vi "Actor Core.vi"(8 "error in":errorcluster, 11 "HIJ 4 Aligment Cams Launcher in":refnum<class "HIJ 4 Aligment Cams Launcher.lvclass">) -> (0 "error out":errorcluster, 3 "Actor out":refnum<class "Actor.lvclass">)   [LabVIEW 2014, in "HIJ 4 Alignment Cams App.lvlib" / "HIJ 4 Aligment Cams Launcher.lvclass"]
doc: "(<B>Filename</B>: Actor Framework.lvlib:Actor.lvclass:Actor Core.vi)\n\nReceives messages to the actor, reacts to them, and initiates any error handling that may shut the actor down.\n\nDescendant classes may override this VI to append parallel tasks for the actor to complete while it handles messages. Overrides use the Call Parent Method node."
uses:
  HIJ 4 Aligment Cams Launcher.lvclass
  <vilib>/ActorFramework/Actor/Actor.lvclass
  <vilib>/userdefined/High Color/IMAQdx.ctl
  HIJ 4 Alignment Cams App/HIJ 4 Alignment Cams App.lvclass
  HIJ Vision Launcher/HIJ Vision Launcher/HIJ Vision Launcher.lvclass/HIJ Vision Launcher.ctl
  Shared Code/Viewable Actor/ViewableActor/ViewableActor.lvclass/ViewableActor.ctl
  HIJ 4 Alignment Cams App/HIJ 4 Alignment Cams App.lvclass/HIJ 4 Alignment Cams App.ctl
  <vilib>/ActorFramework/Actor/Actor.lvclass/Actor.ctl
  <vilib>/ActorFramework/Message Enqueuer/Message Enqueuer.lvclass/Message Enqueuer.ctl
  HIJ 4 Aligment Cams Launcher Messages/Set Sart Cameras Msg/Set Sart Cameras Msg.lvclass/Set Sart Cameras Msg.ctl
  HIJ Vision Launcher/HIJ Vision Launcher/Read HIJ Vision Camera App.vi
  HIJ Vision Launcher/HIJ Vision Launcher/Read Cmd Parameters.vi
  Shared Code/Viewable Actor/ViewableActor/Read Config URL.vi
  HIJ 4 Alignment Cams App/Write Start Camera 4.vi
  HIJ 4 Alignment Cams App/Write Start Camera 3.vi
  HIJ 4 Alignment Cams App/Write Start Camera 2.vi
  HIJ Vision Launcher/HIJ Vision Launcher/Write HIJ Vision Camera App.vi
  <vilib>/ActorFramework/Message Enqueuer/Init from Existing Queue.vi
  <vilib>/ActorFramework/Message Enqueuer/Enqueue.vi
  <vilib>/Utility/config.llb/Read Key (String).vi
  <vilib>/Utility/config.llb/Write Key (String).vi
  <vilib>/ActorFramework/Message Priority Queue/Priority Enqueue.vi
  Shared Code/Viewable Actor/ViewableActor/ViewableActor.lvclass
  <vilib>/ActorFramework/Message Enqueuer/Message Enqueuer.lvclass
  HIJ 4 Aligment Cams Launcher Messages/Set Sart Cameras Msg/Set Sart Cameras Msg.lvclass
  <vilib>/ActorFramework/Stop Msg/Stop Msg.lvclass
  HIJ Vision Launcher/HIJ Vision Launcher/HIJ Vision Launcher.lvclass
  <vilib>/Utility/config.llb/NI_LVConfig.lvlib
panel:
  in  "Camera 2":T1="dummy"
  in  "Camera 3":T1="dummy"
  in  "Main Camera 4":T1="dummy"
  in  "RUN_STOP":bool
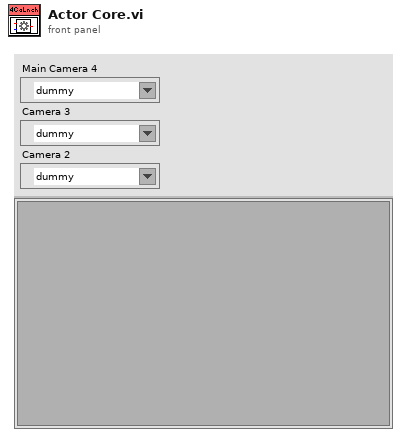
[diagram p1: front panel]
types:
  T1 = typedef "IMAQdx.ctl" = refnum<k21>
  T2 = typedef "NI_LVConfig.lvlib/Config Data RefNum.ctl" = refnum<k1>
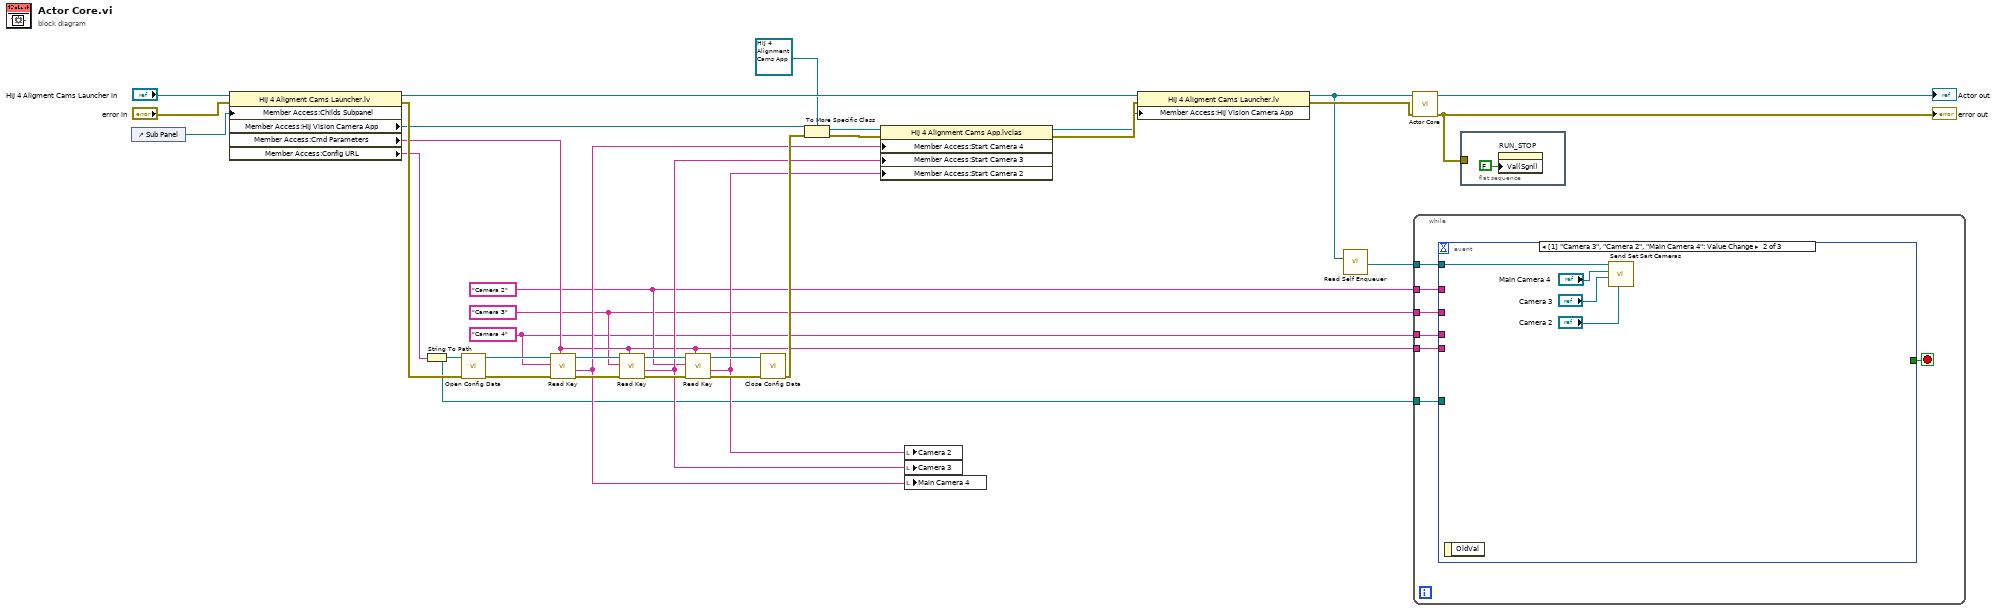
[diagram p0: block diagram]
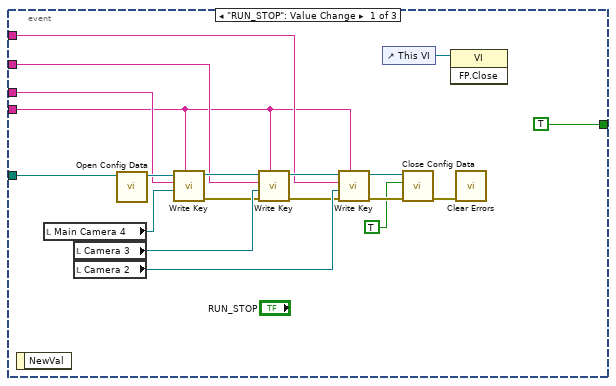
[diagram p2: hidden frame]
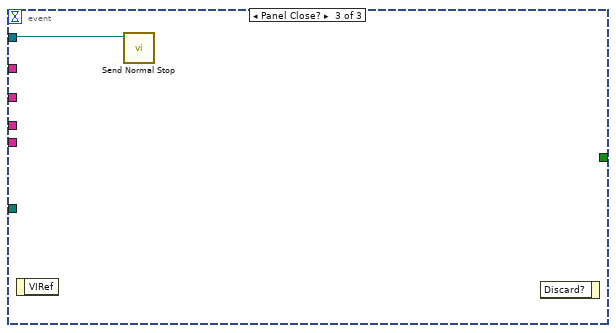
[diagram p3: hidden frame]
diagram:
  w10 = "Camera 2" ("key")
  w9 = "Camera 3" ("key")
  w8 = "Camera 4" ("key")
  n1 = control-ref of="Sub Panel"() -> (w29:refnum<vi>)
  n2 = property class="HIJ 4 Aligment Cams Launcher.lv"(reference="HIJ 4 Aligment Cams Launcher in", error in="error in", "Member Access:Childs Subpanel"=w29) -> (reference out=w30:refnum<class "HIJ 4 Aligment Cams Launcher.lvclass">, error out=w33:errorcluster, "Member Access:HIJ Vision Camera App"=w4:refnum<class "ViewableActor.lvclass">, "Member Access:Cmd Parameters"=w11:string, "Member Access:Config URL"=w28:string)
  n3 = String To Path(string=w28) -> (path=w16:path)
  n4 = call <vilib>:"Open Config Data.vi"("error in (no error)"=w33, "configuration file path"=w16) -> ("error out"=w27:errorcluster, "refnum"=w26:T2)  [unwired: 7 in, 1 out]
  n5 = call-poly <vilib>:"Read Key.vi"("section"=w11, "error in (no error)"=w27, "key"=w8, "refnum"=w26) -> ("error out"=w24:errorcluster, "value"=w19:string, "refnum out"=w25:T2)  [unwired: 4 in, 1 out]
  n6 = call-poly <vilib>:"Read Key.vi"("section"=w11, "error in (no error)"=w24, "key"=w9, "refnum"=w25) -> ("error out"=w22:errorcluster, "value"=w18:string, "refnum out"=w23:T2)  [unwired: 4 in, 1 out]
  n7 = call-poly <vilib>:"Read Key.vi"("section"=w11, "error in (no error)"=w22, "key"=w10, "refnum"=w23) -> ("error out"=w20:errorcluster, "value"=w17:string, "refnum out"=w21:T2)  [unwired: 4 in, 1 out]
  n8 = call <vilib>:"Close Config Data.vi"("error in (no error)"=w20, "refnum"=w21) -> ("error out"=w34:errorcluster)  [unwired: 8 in, 1 out]
  n9 = To More Specific Class(target class=refnum<class "HIJ 4 Alignment Cams App.lvclass"> refnum ("HIJ 4 Alignment Cams App.lvlib:HIJ 4 Alignment Cams App.lvclass"), reference=w4, error in=w34) -> (specific class reference=w1:refnum<class "HIJ 4 Alignment Cams App.lvclass">, error out=w3:errorcluster)
  n10 = property class="HIJ 4 Alignment Cams App.lvclas"(reference=w1, error in=w3, "Member Access:Start Camera 4"=w19, "Member Access:Start Camera 3"=w18, "Member Access:Start Camera 2"=w17) -> (reference out=w2:refnum<class "HIJ 4 Alignment Cams App.lvclass">, error out=w14:errorcluster)
  n11 = local write "Camera 2"(w17) -> ()
  n12 = local write "Camera 3"(w18) -> ()
  n13 = local write "Main Camera 4"(w19) -> ()
  n14 = property class="HIJ 4 Aligment Cams Launcher.lv"(reference=w30, error in=w14, "Member Access:HIJ Vision Camera App"=w2) -> (reference out=w12:refnum<class "HIJ 4 Aligment Cams Launcher.lvclass">, error out=w13:errorcluster)
  n15 = call <vilib>:"Read Self Enqueuer.vi"("Actor"=w12) -> ("Self Enqueuer"=w7:refnum<class "Message Enqueuer.lvclass">)  [unwired: 10 in]
  n16 = call-parent "Actor Core.vi"("error in"=w13, "HIJ Vision Launcher in"=w12) -> ("error out"=w6:errorcluster, "Actor out"=→"Actor out":refnum<class "Actor.lvclass">)  [unwired: 8 in]
  "error out" <- w6
  n17 = while {
    tunnel: w11 -> [w40]
    tunnel: w16 -> [w39]
    tunnel: w8 -> [w38]
    tunnel: w9 -> [w37]
    tunnel: w10 -> [w36]
    tunnel: w7 -> [w35]
    stop <- w41 stop-if-true
    n18 = event shown="[1] \"Camera 3\", \"Camera 2\", \"Main Camera 4\": Value Change" {
      selector: _ -> [_ _ _]
      dyn-events: _ -> [_ _ _]
      timeout: _ -> [_ _ _]
      tunnel: [TRUE _ _] -> w41
      tunnel: w40 -> [w43 _ _]
      tunnel: w39 -> [w48 _ _]
      tunnel: w38 -> [w46 _ _]
      tunnel: w37 -> [w45 _ _]
      tunnel: w36 -> [w44 _ _]
      tunnel: w35 -> [_ w64 w65]
      event "RUN_STOP": Value Change {
        n19 = event-data() -> ()  [unwired: 1 in, 1 out]
        n20 = local read "Main Camera 4"() -> (w53:T1)
        n21 = local read "Camera 3"() -> (w58:T1)
        n22 = local read "Camera 2"() -> (w59:T1)
        n23 = call <vilib>:"Open Config Data.vi"("configuration file path"=w48) -> ("refnum"=w47:T2)  [unwired: 8 in, 2 out]
        n24 = call-poly <vilib>:"Write Key.vi"("section"=w43, "value"=w53, "key"=w46, "refnum"=w47) -> ("error out"=w51:errorcluster, "refnum out"=w52:T2)  [unwired: 5 in, 1 out]
        n25 = call-poly <vilib>:"Write Key.vi"("section"=w43, "error in (no error)"=w51, "value"=w58, "key"=w45, "refnum"=w52) -> ("error out"=w56:errorcluster, "refnum out"=w57:T2)  [unwired: 4 in, 1 out]
        n26 = call-poly <vilib>:"Write Key.vi"("section"=w43, "error in (no error)"=w56, "value"=w59, "key"=w44, "refnum"=w57) -> ("error out"=w55:errorcluster, "refnum out"=w54:T2)  [unwired: 4 in, 1 out]
        n27 = control-ref of="This VI"() -> (w42:refnum<vi>)
        n28 = call <vilib>:"Close Config Data.vi"("error in (no error)"=w55, "write file if changed (T)"=TRUE, "refnum"=w54) -> ("error out"=w49:errorcluster)  [unwired: 7 in, 1 out]
        n29 = invoke class="VI" method="FP.Close"(reference=w42) -> ()  [unwired: 2 in, 3 out]
        n30 = call <vilib>:"Clear Errors.vi"("error in (no error)"=w49) -> ()  [unwired: 5 in, 2 out]
      }
      event Value Change {
        n31 = event-data() -> ()  [unwired: 1 in, 1 out]
        n32 = call "Send Set Sart Cameras.vi"("Camera 2"="Camera 2", "Camera 3"="Camera 3", "Main Camera 4"="Main Camera 4", "Message Enqueuer"=w64) -> ()  [unwired: 6 in, 2 out]
      }
      event Panel Close? {
        n33 = event-data() -> ()  [unwired: 1 in, 1 out]
        n34 = call <vilib>:"Send Normal Stop.vi"("Message Enqueuer"=w65) -> ()  [unwired: 10 in, 1 out]
        n35 = event-data() -> ()  [unwired: 2 in, 1 out]
      }
    }
  }
  n36 = flat-sequence {
    tunnel: w6 -> [_]
    frame #0 {
      n37 = property on="RUN_STOP" class="Bool (strict)"("Val(Sgnl)"=FALSE ("Value (Signaling)")) -> ()  [unwired: 2 in, 2 out]
    }
  }
